vi "respuesta read adc.vi"(8 "error in (no error)":errorcluster, 11 "simulado in":refnum<class "simulado.lvclass">) -> (0 "error out":errorcluster, 2 "salida":string, 3 "simulado out":refnum<class "simulado.lvclass">)   [LabVIEW 2019, in "simulado.lvclass"]
uses:
  simulado.lvclass
  simulado.lvclass/simulado.ctl
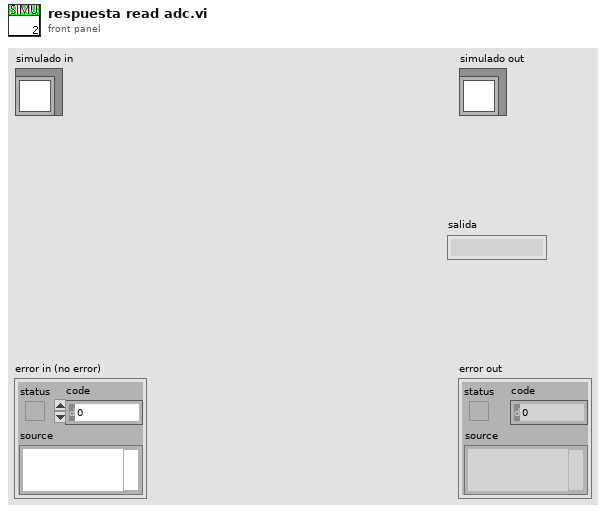
[diagram p1: front panel]
types:
  T1 = enum16{"get parameter", "Set parameters", "reset parameter", ""}
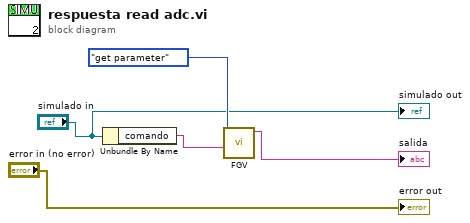
[diagram p0: block diagram]
diagram:
  n1 = Unbundle By Name("simulado in") -> ("comando"=w3:string)
  n2 = call "FGV.vi"("command"=w3, "functions"=T1."get parameter") -> ("response retrirvrd"=→"salida":string)  [unwired: 8 in, 1 out]
  "error out" <- "error in (no error)"
  "simulado out" <- "simulado in"
